vi "Monitor Minimum Samples Ready.vi"(7 "stream.num samples 0":u64, 10 "permissed elements":u32, 11 "stream.minimum elements to start 0":u32) -> (3 "ready for start":bool)   [LabVIEW 2015, in "niInstr Streaming v1 FPGA.lvlib"]
doc: "<b>Monitor Minimum Samples Ready</B> is used to enable the FPGA to independently manage waiting for the FIFO to be primed. It is an optional VI, which is most often useful applications that require uninterrupted streaming output.\n\nA user who would prefer the host to manage waiting for the FIFO to be primed may prefer to use the VI <b>Monitor FIFO Health</b> for the task.\n\nAll terminals with a number suffix are intended to be connected to the host by controls and indicators. The number allows the host to resolve different stream numbers from the host interface. However, this VI does not have a standard VI on the host to program this value. A user may use the stock NI-RIO FPGA Host Interface to write to the controls.\n\n<b>stream.minimum elements to start N</b> is used to specify the minimum number of samples to wait for permission to use before asserting the output <b>ready for start</b> to true.\n\n<b>stream.num samples N</b> should be connected to the same named control used in the <B>Data Stream Control</b> VI. This is to enable the monitor to autonomously choose between the programmed \"minimum\" above and the specified maximum in stream.num samples. This allows a user to specify a transfer size smaller than the \"minimum\" - but still automatically start when all data that will be transferred is ready.\n\n<b>permissed elements</b> \nA user should connect the output of the FPGA FIFO Method \"Get Number of Elements to Read\" or \"Get Number of Elements to Write\" for the FIFO that will be monitored."
uses:
  <instrlib>/_niInstr/Streaming/v1/FPGA/niInstr Streaming v1 FPGA.lvlib
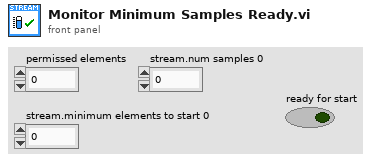
[diagram p1: front panel]
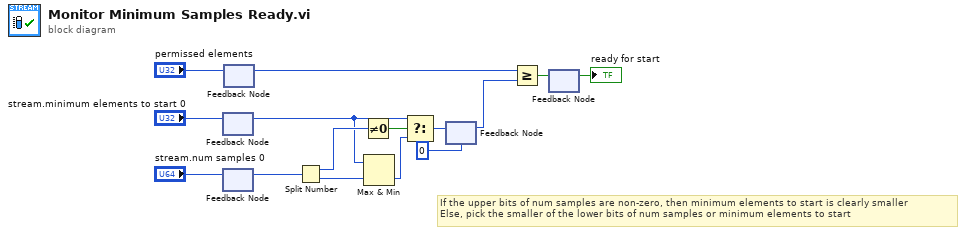
[diagram p0: block diagram]
diagram:
  # "If the upper bits of num samples are non-zero, then minimum elements to start is clearly smaller\nElse, pick the smaller of the lower bits of num samples or minimum elements to start"
  n1 = feedback #1() -> (w4:u32)  [unwired: 1 in]
  n2 = feedback-in #1("stream.minimum elements to start 0") -> ()
  n3 = feedback #2() -> (w6:u64)  [unwired: 1 in]
  n4 = feedback-in #2("stream.num samples 0") -> ()
  n5 = feedback #3() -> (w2:u32)  [unwired: 1 in]
  n6 = feedback-in #3("permissed elements") -> ()
  n7 = Split Number(x=w6) -> (hi(x)=w13:u32, lo(x)=w14:u32)
  n8 = Not Equal To 0?(x=w13) -> (x != 0?=w12:bool)
  n9 = Max & Min(x=w4, y=w14) -> (min(x,y)=w11:u32)  [unwired: 1 out]
  n10 = Select(t=w4, s=w12, f=w11) -> (s? t:f=w10:u32)
  n11 = feedback-in #4(w10) -> ()
  n12 = feedback #4(u32 0 ("stream.minimum elements to start 0")) -> (w9:u32)
  n13 = Greater Or Equal?(x=w2, y=w9) -> (x >= y?=w15:bool)
  n14 = feedback-in #5(w15) -> ()
  n15 = feedback #5() -> (→"ready for start":bool)  [unwired: 1 in]
